vi "Beta 1.2.1.vi"() -> ()   [LabVIEW 2011]
panel:
  out "XY Graph":cluster{dbl[], dbl[]}(graph)
  out "Original Image":T1(plugin-control)
  out "Path to Image":path
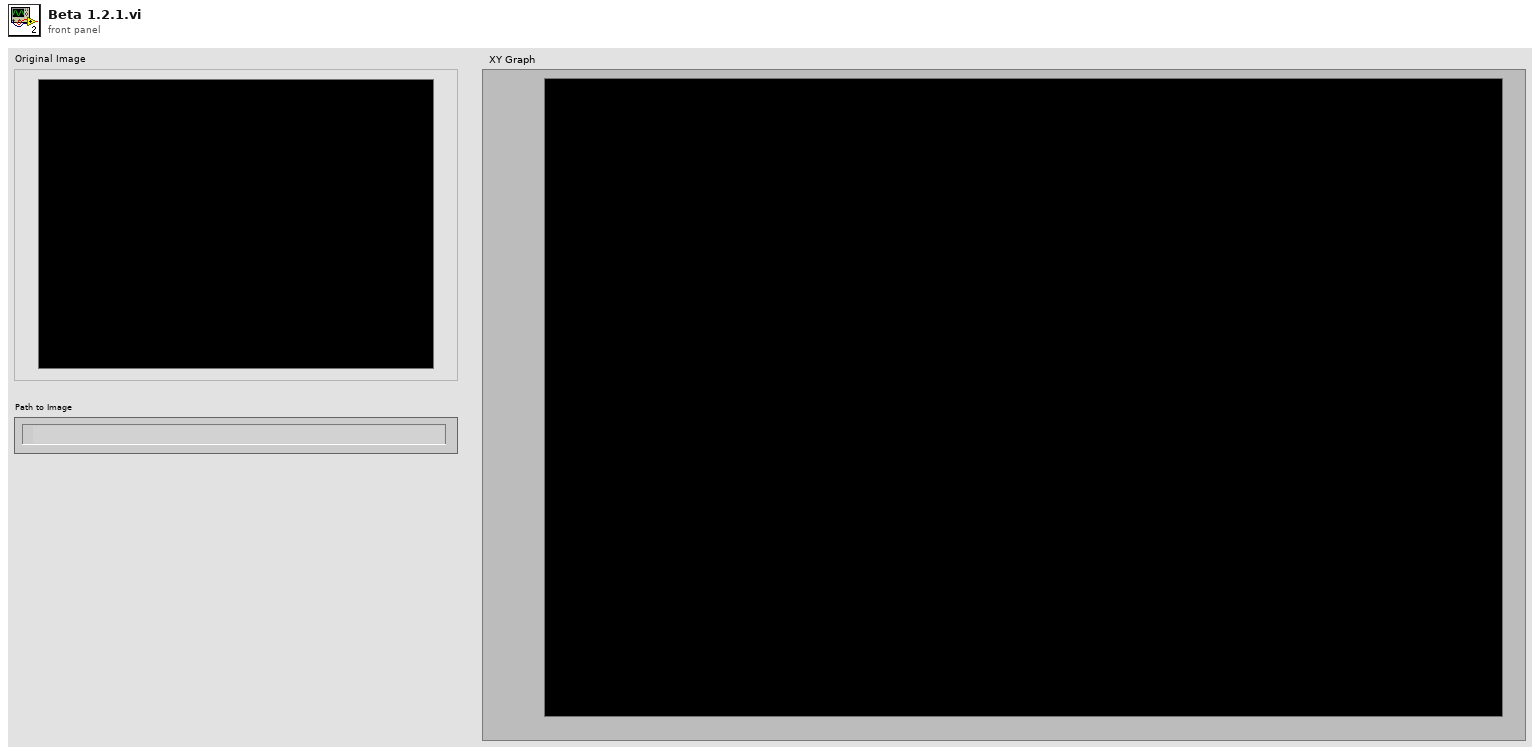
[diagram p1: front panel]
types:
  T1 = typedef "IMAQ Image.ctl" = refnum<image>
  T2 = typedef "Image Type" = u32
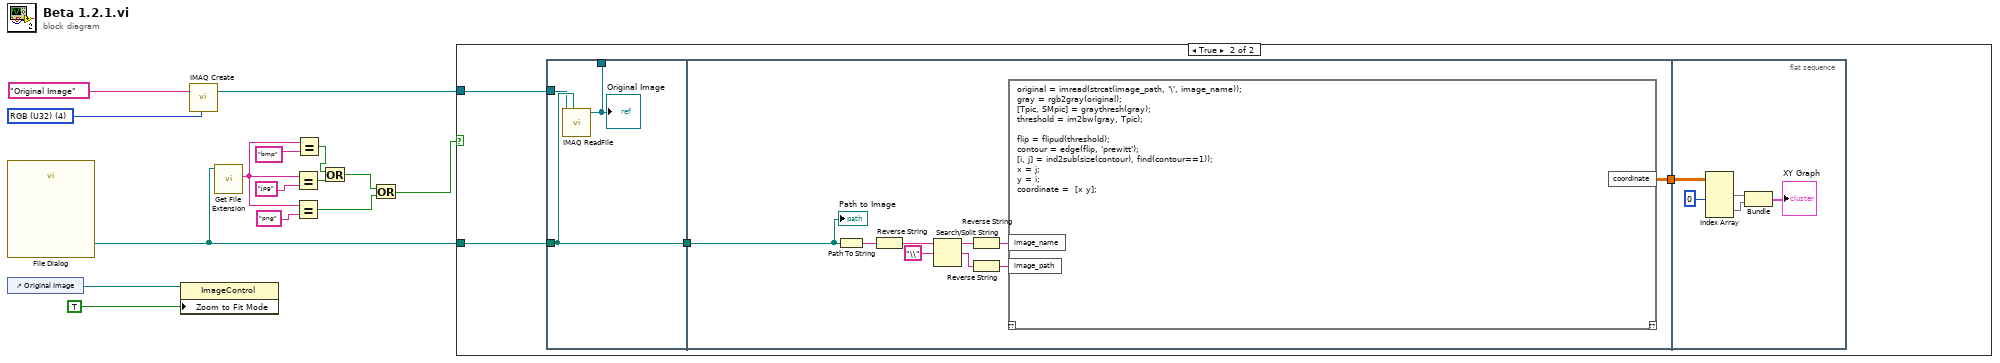
[diagram p0: block diagram]
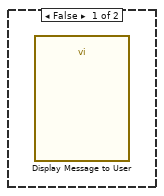
[diagram p2: hidden frame]
diagram:
  w14 = T2 4 items=["Grayscale (U8)", "Grayscale (I16)", "Grayscale (SGL)", "Complex (CSG)", "RGB (U32)", "HSL (U32)", "RGB (U64)", "Grayscale (U16)"] ("Image Type")
  n1 = call "File Dialog"() -> ("selected path"=w10:path)  [unwired: 12 in, 3 out]
  n2 = control-ref of="Original Image"() -> (w12:refnum<vi>)
  n3 = property class="ImageControl"(reference=w12, "Zoom to Fit Mode"=TRUE) -> ()  [unwired: 1 in, 2 out]
  n4 = call "IMAQ Create"("Image Name"="Original Image", "Image Type"=w14) -> ("New Image"=w13:T1)  [unwired: 3 in, 1 out]
  n5 = call <vilib>:"Get File Extension.vi"("file"=w10) -> ("lowercase file extension"=w8:string)  [unwired: 7 in, 3 out]
  n6 = Equal?(x=w8, y="jpg") -> (x = y?=w4:bool)
  n7 = Equal?(x=w8, y="png") -> (x = y?=w2:bool)
  n8 = Equal?(x=w8, y="bmp") -> (x = y?=w5:bool)
  n9 = Or(x=w5, y=w4) -> (x .or. y?=w3:bool)
  n10 = Or(x=w3, y=w2) -> (x .or. y?=w1:bool)
  n11 = case shown="True" w1 {
    tunnel: w10 -> [_ w17]
    tunnel: w13 -> [_ w16]
    frame False {
      n12 = call "Display Message to User"() -> ()  [unwired: 10 in, 2 out]
    }
    frame True {
      n13 = flat-sequence {
        tunnel: [w21] -> w19
        tunnel: [w22] -> _
        tunnel: w17 -> [w21]
        tunnel: w16 -> [w20]
        tunnel: w19 -> [w23]
        tunnel: [w24] -> w18
        tunnel: w18 -> [w36]
        frame #0 {
          n14 = call "IMAQ ReadFile"("File Path"=w21, "Image"=w20) -> ("Image Out"=w22:T1)  [unwired: 5 in, 4 out]
          "Original Image" <- w22
        }
        frame #1 {
          n15 = Path To String(path=w23) -> (string=w31:string)
          n16 = Reverse String(1:w31) -> (0:w30:string)
          n17 = Search/Split String(string=w30, search string/char (-)="\\") -> (substring before match=w28:string, match + rest of string=w27:string)  [unwired: 1 in, 1 out]
          n18 = Reverse String(1:w28) -> (0:w26:string)
          n19 = Reverse String(1:w27) -> (0:w25:string)
          n20 = script code="original = imread(strcat(image_path, '\\', image_name));\ngray = rgb2gray(original);\n[Tpic, SMpic] = graythresh(gray);\nthreshold = im2bw(gray, Tpic);\n\nflip = flipud(threshold);\ncontour = edge(flip, 'prewitt');\n[i, j] = ind2sub(size(contour), find(contour==1));\nx = j;\ny = i;\ncoordinate =  [x y];"("image_name"=w26, "image_path"=w25) -> ("coordinate"=w24:dbl[][])  [unwired: 1 in, 1 out]
          "Path to Image" <- w23
        }
        frame #2 {
          n21 = Index Array(array=w36, index (col) #1=0 ("disabled index (col)")) -> (element #1=w34:dbl[], element #2=w33:dbl[])  [unwired: 3 in]
          n22 = Bundle(w34, w33) -> (→"XY Graph":cluster{dbl[], dbl[]})  [unwired: 1 in]
        }
      }
    }
  }
